vi "TEST - Array to Set - Set to Array.vi"(8 "error in":errorcluster) -> (0 "error out":errorcluster, 2 "Pass?":bool)   [LabVIEW 2020, in "test_openg_array.lvlib"]
uses:
  8102667c-31a8-4bac-a57a-145832b45d8f.vi
  8102667c-31a8-4bac-a57a-145832b45d8f.vi/7c7783df-fd5a-49d9-9b7a-63cc9fb0e4e5.vi
  source/library/Get Collection Subtype.vi
  <vilib>/addons/_JKI Toolkits/Caraya/classes/Assert/Assert True.vi
  test_openg_array.lvlib
  source/library/openg_variant.lvlib
  <vilib>/addons/_JKI Toolkits/Caraya/classes/Test/Test.lvclass
  <vilib>/addons/_JKI Toolkits/Caraya/classes/Assert/Assert.lvclass
panel:
  out "Pass (Array to Set)?":bool
  out "Pass (Set to Array)?":bool
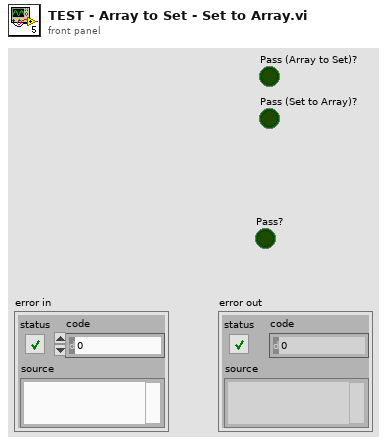
[diagram p1: front panel]
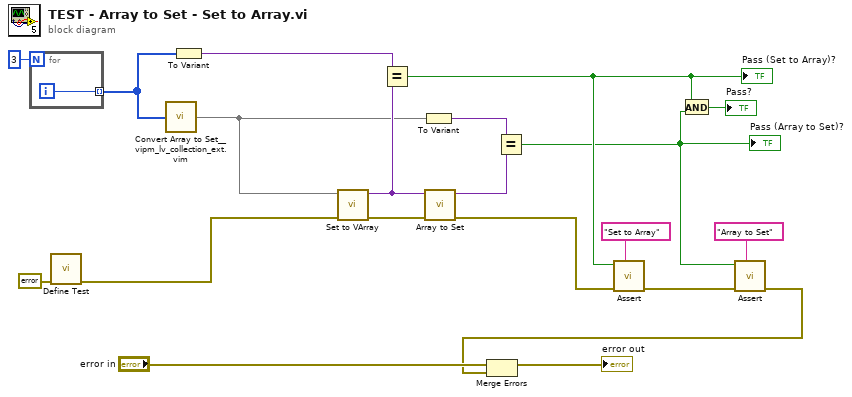
[diagram p0: block diagram]
diagram:
  n1 = for {
    N: 3 -> [_]
    tunnel: [w21] -> w19 mode=indexing
    i -> [w21]
  }
  n2 = call <vilib>:"Define Test.vi"("error in (no error)"=errorcluster {"status"=FALSE, "code"=0, "source"=""}) -> ("error out"=w8:errorcluster)  [unwired: 9 in, 1 out]
  n3 = call "Convert Array to Set__vipm_lv_collection_ext.vim"("array"=w19) -> ("set"=w14:set{i32})  [unwired: 6 in]
  n4 = To Variant(anything=w19) -> (Variant=w18:variant)
  n5 = call "Set to VArray.vi"("error in"=w8, "Set"=w14) -> ("error out"=w10:errorcluster, "Array"=w17:variant)  [unwired: 8 in]
  n6 = Equal?(x=w18, y=w17) -> (x = y?=w6:bool)
  "Pass (Set to Array)?" <- w6
  n7 = To Variant(anything=w14) -> (Variant=w15:variant)
  n8 = call "Array to Set.vi"("error in"=w10, "Array"=w17) -> ("error out"=w7:errorcluster, "Set"=w16:variant)  [unwired: 8 in]
  n9 = Equal?(x=w15, y=w16) -> (x = y?=w5:bool)
  "Pass (Array to Set)?" <- w5
  n10 = call-poly <vilib>:"Assert.vi"("Label"="Set to Array" ("Label (VI Title)"), "error in (no error)"=w7, "True?"=w6) -> ("error out"=w9:errorcluster)  [unwired: 7 in, 1 out]
  n11 = And(x=w6, y=w5) -> (x .and. y?=→"Pass?":bool)
  n12 = call-poly <vilib>:"Assert.vi"("Label"="Array to Set" ("Label (VI Title)"), "error in (no error)"=w9, "True?"=w5) -> ("error out"=w1:errorcluster)  [unwired: 7 in, 1 out]
  n13 = Merge Errors("error in", w1) -> (→"error out":errorcluster)
